vi "State Exit.vi"(8 "error in (no error)":errorcluster, 11 "View Model":T1) -> (0 "error out":errorcluster, 3 "View Model":T1)   [LabVIEW 2017]
doc: "Handle state transitions"
uses:
  View Model/Controls/View Model.ctl
  Error Handler/Controls/Error Model.ctl
  Error Handler/Controls/Error Type.ctl
  View Model/Controls/Shared Model.ctl
  Controls/Elevator Model.ctl
  Controls/Controller Overhead.ctl
  Controls/Elevator Commands.ctl
  Configuration/Controls/Configuration Model.ctl
  Configuration/Controls/Configuration Data.ctl
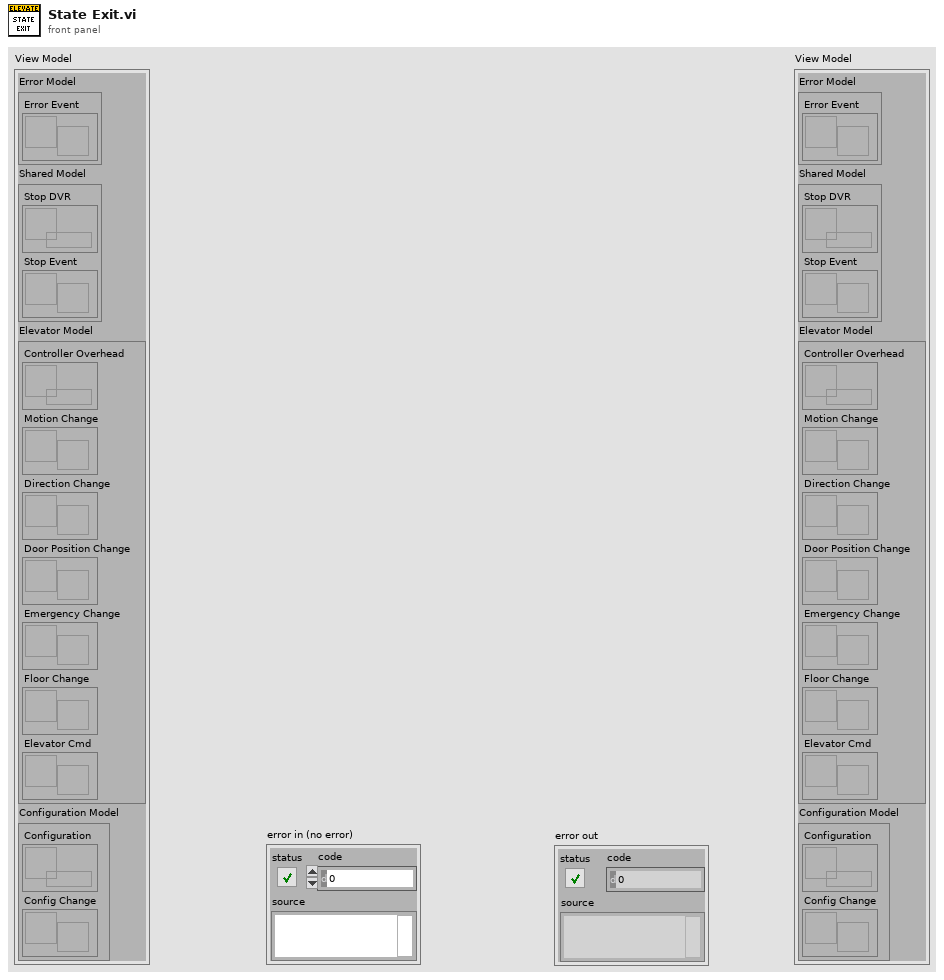
[diagram p1: front panel]
types:
  T1 = typedef "View Model.ctl" = cluster{"Error Model":T2, "Shared Model":T3, "Elevator Model":T4, "Configuration Model":T5}
  T2 = typedef "Error Model.ctl" = cluster{"Error Event":refnum<user-event>}
  T3 = typedef "Shared Model.ctl" = cluster{"Stop DVR":refnum<data-value>, "Stop Event":refnum<user-event>}
  T4 = typedef "Elevator Model.ctl" = cluster{"Controller Overhead":refnum<data-value>, "Motion Change":refnum<user-event>, "Direction Change":refnum<user-event>, "Door Position Change":refnum<user-event>, "Emergency Change":refnum<user-event>, "Floor Change":refnum<user-event>, "Elevator Cmd":refnum<user-event>}
  T5 = typedef "Configuration Model.ctl" = cluster{"Configuration":refnum<data-value>, "Config Change":refnum<user-event>}
  T6 = enum16{"Idle", "Open Doors", "Close Doors", "Start Move", "Move", "Finish Move", "Emergency"}
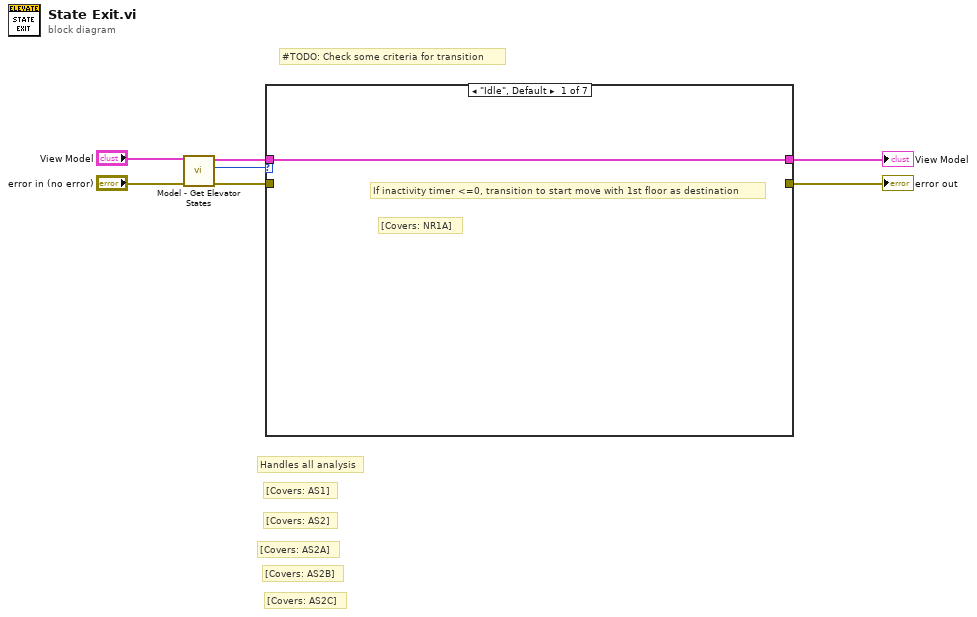
[diagram p0: block diagram]
diagram:
  # "[Covers: AS2C]"
  # "[Covers: AS2B]"
  # "[Covers: AS2A]"
  # "[Covers: AS2]"
  # "[Covers: AS1]"
  # "Handles all analysis"
  # "#TODO: Check some criteria for transition"
  n1 = call "Model - Get Elevator States.vi"("error in (no error)"="error in (no error)", "View Model"="View Model") -> ("error out"=w2:errorcluster, "Elevator State"=w6:T6, "View Model"=w5:T1)  [unwired: 6 in, 1 out]
  n2 = case shown="\"Idle\", Default" w6 {
    tunnel: w5 -> [w8 w10 w11 w12 w13 w14 w15]
    tunnel: [w8 w10 w11 w12 w13 w14 w15] -> w4
    tunnel: w2 -> [_ w9 _ _ _ _ _]
    tunnel: [_ w9 _ _ _ _ _] -> w1
    frame "Idle", Default {
      # "[Covers: NR1A]"
      # "If inactivity timer <=0, transition to start move with 1st floor as destination"
    }
    frame "Open Doors" {
      # "[Covers: OC3B]"
      # "If open door timer <=0, go to close state"
    }
    frame "Close Doors" {
      # "[Covers: OC7]"
      # "Transition to initial state"
    }
    frame "Start Move" {
    }
    frame "Emergency" {
    }
    frame "Move" {
      # "[Covers: CT1B]"
      # "[Covers: SS4B]"
      # "If time has elapsed, stop elevator. Update floor position"
    }
    frame "Finish Move" {
      # "[Covers: RF3]"
      # "Transition to door open/close"
    }
  }
  "error out" <- w1
  "View Model" <- w4
